vi "WMI_GetInstalledPrinters.vi"(8 "error in (no error)":errorcluster) -> (0 "error out":errorcluster, 1 "IsDefaultPrinter":bool[](array[boolean]), 2 "NetworkPrinter":bool[](array[boolean]), 3 "Names":string[](array[string]), 4 "Count":i32, 5 "Status":string[](array[string]))   [LabVIEW 2021, in "LUGE_2022.4.lvlib"]
doc: "Returns the list of installed printers on this computer.\nReturns also, a status, if the printer is available through the network and if it's the default printer."
uses:
  System.Management
  LUGE_2022.4.lvlib
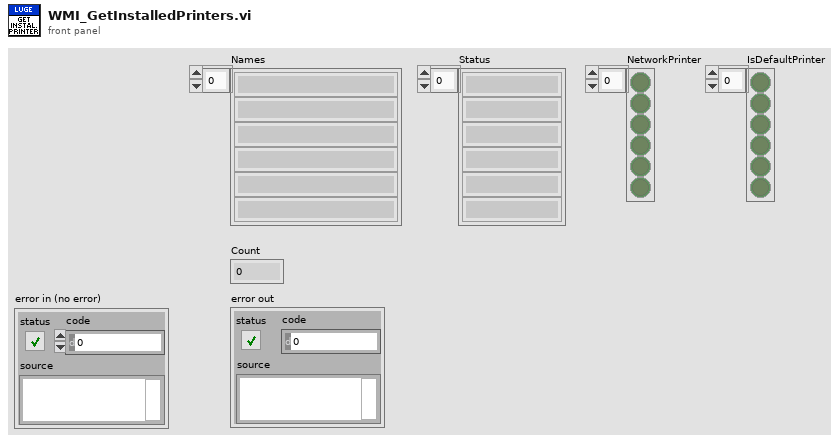
[diagram p1: front panel]
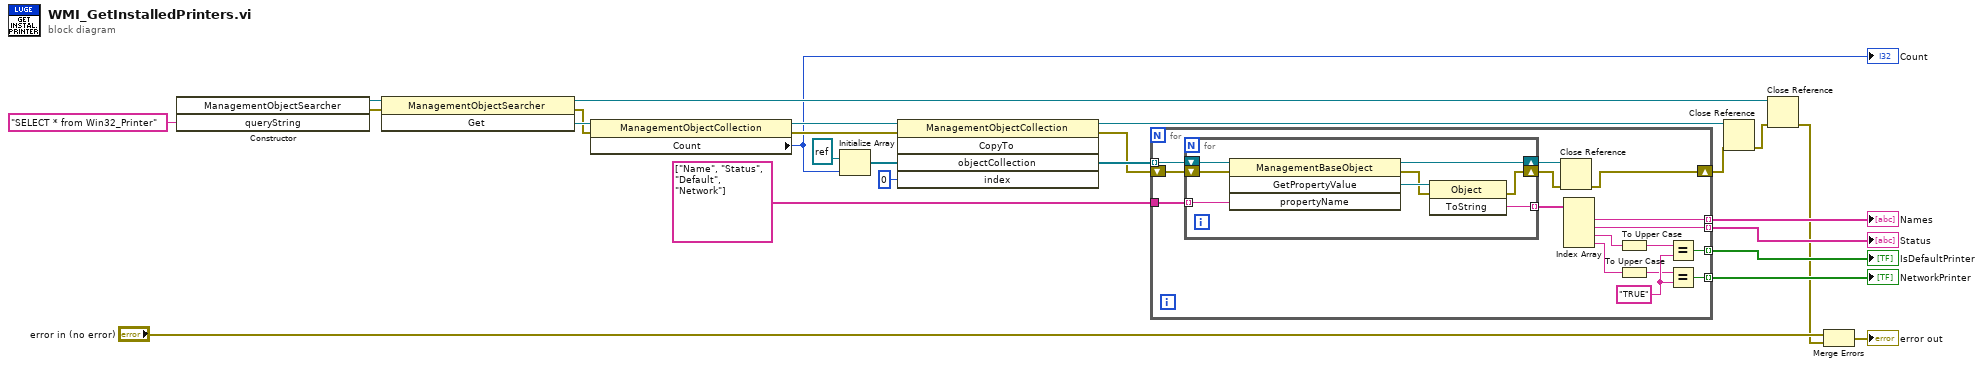
[diagram p0: block diagram]
diagram:
  n1 = constructor class="ManagementObjectSearcher"("queryString"="SELECT * from Win32_Printer" ("scope")) -> (reference out=w24:refnum<k24>, error out=w23:errorcluster)  [unwired: 3 in, 2 out]
  n2 = invoke class="ManagementObjectSearcher" method="Get"(reference=w24, error in=w23) -> (reference out=w20:refnum<k24>, error out=w21:errorcluster, "Get"=w22:refnum<k24>)  [unwired: 1 in]
  n3 = property class="ManagementObjectCollection"(reference=w22, error in=w21) -> (reference out=w6:refnum<k24>, error out=w7:errorcluster, "Count"=w2:i32)
  "Count" <- w2
  n4 = Initialize Array(refnum<k24> refnum ("element"), w2) -> (w9:refnum<k24>[])
  n5 = invoke class="ManagementObjectCollection" method="CopyTo"(reference=w6, error in=w7, "objectCollection"=w9, "index"=0) -> (reference out=w3:refnum<k24>, error out=w4:errorcluster, "objectCollection"=w5:refnum<k24>[])  [unwired: 1 in, 2 out]
  n6 = for {
    tunnel: string[] ["Name", "Status", "Default", "Network"] -> [w41]
    tunnel: [w37] -> w15 mode=indexing
    tunnel: [w36] -> w14 mode=indexing
    tunnel: [w30] -> w16 mode=indexing
    tunnel: [w29] -> w17 mode=indexing
    tunnel: w5 -> [w26] mode=indexing
    shift-right: [w27] -> w1
    shift-left: w4 -> [w28]
    w33 = "TRUE"
    n7 = for {
      tunnel: w41 -> [w46] mode=indexing
      tunnel: [w45] -> w38 mode=indexing
      shift-right: [w43] -> w40
      shift-left: w26 -> [w49]
      shift-right: [w42] -> w39
      shift-left: w28 -> [w48]
      n8 = invoke class="ManagementBaseObject" method="GetPropertyValue"(reference=w49, error in=w48, "propertyName"=w46) -> (reference out=w43:refnum<k24>, error out=w44:errorcluster, "GetPropertyValue"=w47:refnum<k24>)  [unwired: 1 in, 1 out]
      n9 = invoke class="Object" method="ToString"(reference=w47, error in=w44) -> (error out=w42:errorcluster, "ToString"=w45:string)  [unwired: 1 in, 1 out]
    }
    n10 = Close Reference(reference=w40, error in (no error)=w39) -> (error out=w27:errorcluster)
    n11 = Index Array(array=w38) -> (element #1=w37:string, element #2=w36:string, element #3=w35:string, element #4=w34:string)  [unwired: 4 in]
    n12 = To Upper Case(1:w35) -> (0:w31:string)
    n13 = To Upper Case(1:w34) -> (0:w32:string)
    n14 = Equal?(x=w31, y=w33) -> (x = y?=w30:bool)
    n15 = Equal?(x=w32, y=w33) -> (x = y?=w29:bool)
  }
  "NetworkPrinter" <- w17
  "IsDefaultPrinter" <- w16
  "Names" <- w15
  "Status" <- w14
  n16 = Close Reference(reference=w3, error in (no error)=w1) -> (error out=w18:errorcluster)
  n17 = Close Reference(reference=w20, error in (no error)=w18) -> (error out=w12:errorcluster)
  n18 = Merge Errors("error in (no error)", w12) -> (→"error out":errorcluster)
